vi "AAA Waveform, Catalog.vi"   [LabVIEW 2010]
uses:
  Waveform Attribute/Waveform Attribute Cluster.ctl
panel:
  # "Waveform\nCatalog"
types:
  T1 = typedef "Waveform Attribute Cluster.ctl" = cluster{"Label":string, "Value":dbl}
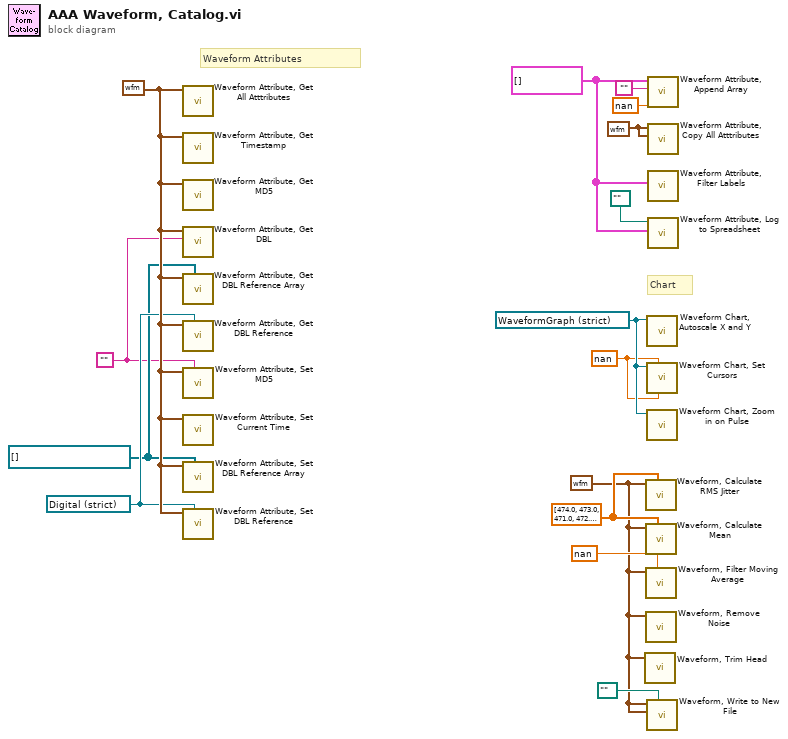
[diagram p0: block diagram]
diagram:
  w3 = dbl[] [474.0, 473.0, 471.0, 472.0, 473.0, 473.0, 473.0] ("index")
  w1 = waveform(dbl) {"t0"=timestamp(3473168117.0530005 s since 1904-01-01), "dt"=4e-06, "Y"=array[750000 elements], "attributes"=variant("Average Size"=variant(dbl 15.0), "Frequency (Hz)"=variant(dbl 1.998745962823557), "Number of Samples"=variant(dbl 750000.0), "Process Timestamp"=variant(timestamp timestamp(3474401815.53125 s since 1904-01-01)), "Recvy Amp (V)"=variant(dbl 5.120123508943166), "Recvy Amp (mA)"=variant(dbl 10.240247017886333), "Recvy Frequency (Hz)"=variant(dbl 1.9987453162428834), "Recvy Pulse Width (us)"=variant(dbl 422.33480072021484), "Recvy Trigger (s)"=variant(dbl 0.35626399999999997), "Resistance (ohms)"=variant(dbl 500.0), "Sample Frequency (MHz)"=variant(dbl 0.25), "Stim Amp (V)"=variant(dbl -4.84918832438602), "Stim Amp (mA)"=variant(dbl -9.698376648772038), "Stim Frequency (Hz)"=variant(dbl 1.9987466094042308), "Stim Pulse Width (us)"=variant(dbl 417.8791389465332), "Stim Trigger (s)"=variant(dbl 0.355772), "dt (us)"=variant(dbl 4.0))} ("waveform")
  w5 = nan ("value")
  w8 = T1[] [] ("attributes")
  w10 = ""
  w11 = refnum<vi>[] [] ("Refnum Array")
  w13 = refnum<vi> refnum ("WFGraph ref")
  w12 = refnum<vi> refnum ("Digital DBL Refnum")
  w14 = waveform(dbl) {"t0"=timestamp(3473168117.0530005 s since 1904-01-01), "dt"=4e-06, "Y"=array[750000 elements], "attributes"=variant("Average Size"=variant(dbl 15.0), "Frequency (Hz)"=variant(dbl 1.998745962823557), "Number of Samples"=variant(dbl 750000.0), "Process Timestamp"=variant(timestamp timestamp(3474401815.53125 s since 1904-01-01)), "Recvy Amp (V)"=variant(dbl 5.120123508943166), "Recvy Amp (mA)"=variant(dbl 10.240247017886333), "Recvy Frequency (Hz)"=variant(dbl 1.9987453162428834), "Recvy Pulse Width (us)"=variant(dbl 422.33480072021484), "Recvy Trigger (s)"=variant(dbl 0.35626399999999997), "Resistance (ohms)"=variant(dbl 500.0), "Sample Frequency (MHz)"=variant(dbl 0.25), "Stim Amp (V)"=variant(dbl -4.84918832438602), "Stim Amp (mA)"=variant(dbl -9.698376648772038), "Stim Frequency (Hz)"=variant(dbl 1.9987466094042308), "Stim Pulse Width (us)"=variant(dbl 417.8791389465332), "Stim Trigger (s)"=variant(dbl 0.355772), "dt (us)"=variant(dbl 4.0))} ("waveform")
  w15 = waveform(dbl) {"t0"=timestamp(3473168117.0530005 s since 1904-01-01), "dt"=4e-06, "Y"=array[750000 elements], "attributes"=variant("Average Size"=variant(dbl 15.0), "Frequency (Hz)"=variant(dbl 1.998745962823557), "Number of Samples"=variant(dbl 750000.0), "Process Timestamp"=variant(timestamp timestamp(3474401815.53125 s since 1904-01-01)), "Recvy Amp (V)"=variant(dbl 5.120123508943166), "Recvy Amp (mA)"=variant(dbl 10.240247017886333), "Recvy Frequency (Hz)"=variant(dbl 1.9987453162428834), "Recvy Pulse Width (us)"=variant(dbl 422.33480072021484), "Recvy Trigger (s)"=variant(dbl 0.35626399999999997), "Resistance (ohms)"=variant(dbl 500.0), "Sample Frequency (MHz)"=variant(dbl 0.25), "Stim Amp (V)"=variant(dbl -4.84918832438602), "Stim Amp (mA)"=variant(dbl -9.698376648772038), "Stim Frequency (Hz)"=variant(dbl 1.9987466094042308), "Stim Pulse Width (us)"=variant(dbl 417.8791389465332), "Stim Trigger (s)"=variant(dbl 0.355772), "dt (us)"=variant(dbl 4.0))} ("waveform")
  # "Waveform Attributes"
  # "Chart"
  n1 = call "Waveform Attribute, Get All Atttributes.vi"("waveform"=w15) -> ()  [unwired: 6 in, 3 out]
  n2 = call "Waveform Attribute, Get Timestamp.vi"("waveform"=w15) -> ()  [unwired: 5 in, 4 out]
  n3 = call "Waveform Attribute, Get MD5.vi"("waveform"=w15) -> ()  [unwired: 6 in, 3 out]
  n4 = call "Waveform Attribute, Get DBL.vi"("label"=w10, "waveform"=w15) -> ()  [unwired: 4 in, 4 out]
  n5 = call "Waveform Attribute, Get DBL Reference Array.vi"("refnum array"=w11, "waveform"=w15) -> ()  [unwired: 3 in, 5 out]
  n6 = call "Waveform Attribute, Get DBL Reference.vi"("DigNum Refnum"=w12, "waveform"=w15) -> ()  [unwired: 3 in, 5 out]
  n7 = call "Waveform Attribute, Set MD5.vi"("MD5"=w10, "waveform"=w15) -> ()  [unwired: 6 in, 2 out]
  n8 = call "Waveform Attribute, Set Current Time.vi"("waveform"=w15) -> ()  [unwired: 5 in, 4 out]
  n9 = call "Waveform Attribute, Set DBL Reference Array.vi"("Refnum Array"=w11, "waveform"=w15) -> ()  [unwired: 6 in, 2 out]
  n10 = call "Waveform Attribute, Set DBL Reference.vi"("Digital DBL Refnum"=w12, "waveform"=w15) -> ()  [unwired: 6 in, 2 out]
  n11 = call "Waveform, Trim Head.vi"("waveform"=w1) -> ()  [unwired: 7 in, 3 out]
  n12 = call "Waveform, Calculate RMS Jitter.vi"("waveform"=w1, "transition index"=w3) -> ()  [unwired: 5 in, 4 out]
  n13 = call "Waveform, Calculate Mean.vi"("waveform"=w1, "index"=w3) -> ()  [unwired: 6 in, 3 out]
  n14 = call "Waveform, Filter Moving Average.vi"("Average Size"=nan ("value"), "waveform"=w1) -> ()  [unwired: 6 in, 2 out]
  n15 = call "Waveform, Remove Noise.vi"("waveform"=w1) -> ()  [unwired: 8 in, 2 out]
  n16 = call "Waveform Chart, Autoscale X and Y.vi"("WFGraph ref"=w13) -> ()  [unwired: 9 in, 2 out]
  n17 = call "Waveform Chart, Set Cursors.vi"("PosY"=w5, "PosX"=w5, "WFGraph ref"=w13) -> ()  [unwired: 6 in, 3 out]
  n18 = call "Waveform Chart, Zoom in on Pulse.vi"("WFGraph ref"=w13) -> ()  [unwired: 9 in, 2 out]
  n19 = call "Waveform, Write to New File.vi"("filepath"=path "" ("directory path"), "prc waveform"=w1, "raw waveform"=w1) -> ()  [unwired: 3 in, 4 out]
  n20 = call "Waveform Attribute, Append Array.vi"("value"=nan, "label"="", "attributes"=w8) -> ()  [unwired: 5 in, 2 out]
  n21 = call "Waveform Attribute, Copy All Atttributes.vi"("src waveform"=w14, "dst waveform"=w14) -> ()  [unwired: 4 in, 4 out]
  n22 = call "Waveform Attribute, Filter Labels.vi"("attributes"=w8) -> ()  [unwired: 7 in, 2 out]
  n23 = call "Waveform Attribute, Log to Spreadsheet.vi"("attributes"=w8, "results file"=path "" ("directory path")) -> ()  [unwired: 5 in, 3 out]
